vi "Set Cell Value.vi"(7 "值":string, 8 "error in (no error)":errorcluster caption="错误输入（无错误）", 9 "Y索引":i32, 10 "X索引":i32, 11 "Table Ref In":refnum<vi>) -> (0 "error out":errorcluster caption="错误输出", 3 "Table Ref Out":refnum<vi>)   [LabVIEW 2013, in "Table Tool.lvlib"]
uses:
  Table Tool.lvlib
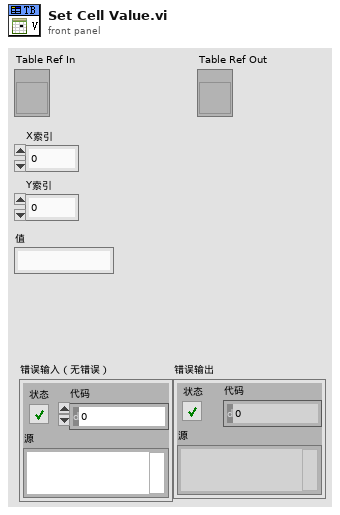
[diagram p1: front panel]
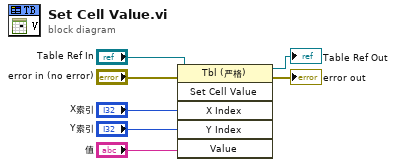
[diagram p0: block diagram]
diagram:
  n1 = invoke class="Tbl (严格)" method="Set Cell Value"(reference="Table Ref In", error in="error in (no error)", "X Index"="X索引", "Y Index"="Y索引", "Value"="值") -> (reference out=→"Table Ref Out":refnum<vi>, error out=→"error out":errorcluster)  [unwired: 1 in, 4 out]
